vi "Constructor.vi"(8 "error in (no error)":errorcluster, 11 "Configuration in":refnum<class "Configuration.lvclass">) -> (0 "error out":errorcluster, 3 "Configuration out":refnum<class "Configuration.lvclass">)   [LabVIEW 2011, in "Configuration.lvclass"]
uses:
  Configuration.lvclass
  Configuration.lvclass/Configuration.ctl
  <vilib>/Utility/config.llb/NI_LVConfig.lvlib
panel:
  out "file created?":bool
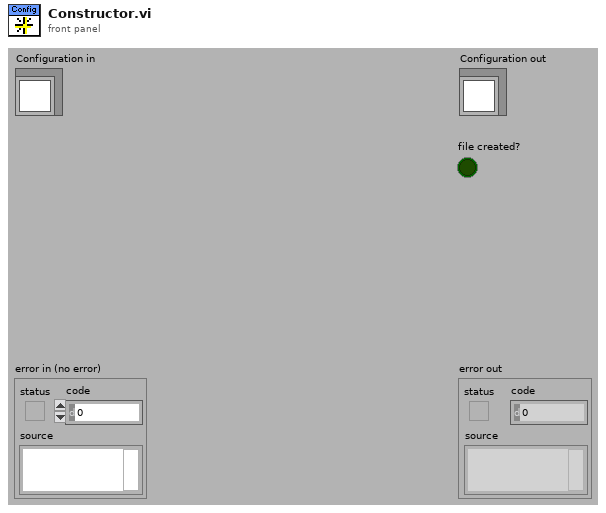
[diagram p1: front panel]
types:
  T1 = typedef "Configuration.lvclass/File Type.ctl" = enum16{"INI", "XML"}
  T2 = typedef "NI_LVConfig.lvlib/Config Data RefNum.ctl" = refnum<k1>
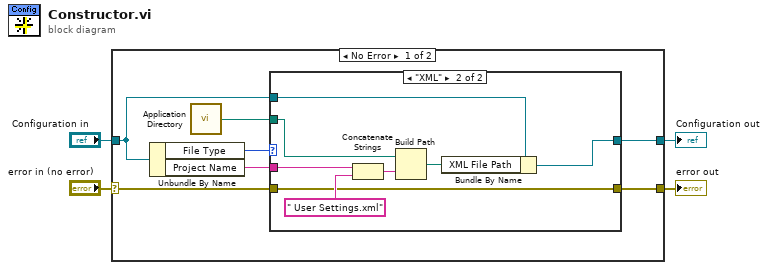
[diagram p0: block diagram]
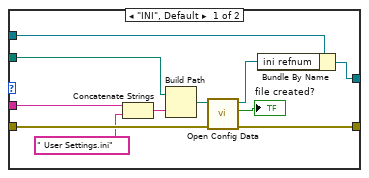
[diagram p2: hidden frame]
diagram:
  n1 = case shown="No Error" "error in (no error)" {
    selector: "error in (no error)" -> [w11 w32]
    tunnel: [w10 w32] -> w3
    tunnel: [w9 w31] -> w1
    tunnel: "Configuration in" -> [w7 w31]
    frame No Error {
      n2 = Unbundle By Name(w7) -> ("File Type"=w8:T1, "Project Name"=w6:string)
      n3 = call <vilib>:"Application Directory.vi"() -> ("Application Directory"=w5:path)
      n4 = case shown="\"XML\"" w8 {
        tunnel: w11 -> [w22 w24]
        tunnel: [w21 w24] -> w10
        tunnel: w7 -> [w20 w27]
        tunnel: [w18 w26] -> w9
        tunnel: w6 -> [w16 w30]
        tunnel: w5 -> [w12 w23]
        frame "INI", Default {
          n5 = Concatenate Strings(w16, " User Settings.ini" ("string")) -> (w14:string)
          n6 = Build Path(base path=w12, name or relative path=w14) -> (appended path=w17:path)
          n7 = call <vilib>:"Open Config Data.vi"("error in (no error)"=w22, "configuration file path"=w17) -> ("error out"=w21:errorcluster, "file created?"=→"file created?":bool, "refnum"=w19:T2)  [unwired: 7 in]
          n8 = Bundle By Name(cluster=w20, "ini refnum"=w19) -> (w18:refnum<class "Configuration.lvclass">)
        }
        frame "XML" {
          n9 = Concatenate Strings(w30, " User Settings.xml" ("string")) -> (w28:string)
          n10 = Build Path(base path=w23, name or relative path=w28) -> (appended path=w25:path)
          n11 = Bundle By Name(cluster=w27, "XML File Path"=w25) -> (w26:refnum<class "Configuration.lvclass">)
        }
      }
    }
    frame Error {
    }
  }
  "error out" <- w3
  "Configuration out" <- w1
